vi "Value Change_Tools.vi"(8 "error in":errorcluster, 10 "NewVal":T8=enum."Ellipse", 11 "Data in":T1={"Class"={"Ants"=refnum, "Layer"=refnum, "Templates"=refnum, "Icon"=refnum, "Glyph"=refnum, "Settings"=refnum, "Tools"=refnum}, "Ref"={"Add Layer"=refnum, "Remove Layer"=refnum, "Line Text"=[], "Body Text Spec"=refnum, "DNL_Font"=refnum, "glyph path str"=refnum, "templates path str"=refnum, "Arrow Up"=refnum, "Arrow Down"=refnum, "IE VI Ref"=refnum, "Glyphs tree"=refnum, "Templates tree"=refnum, "Layer Icon Text"=refnum, "Layer Template"=refnum, "Clipboard"=refnum, "BW icon in"=refnum, "Color icon in"=refnum, "Layer Clust"=refnum, "Body Text"=refnum, "DNL_Framework Templates"=refnum, "Search Templates"=refnum, "TextMarker"=refnum, "Tab Control"=refnum, "Search Glyphs"=refnum, "Line Color"=refnum, "DNL_Glyphs []"=refnum, "Fill Color"=refnum, "Tools"=refnum, "Glyphs tree"=refnum, "Icon"=refnum, "Preview"=refnum, "Ants"=refnum, "Terminals"=refnum, "menu reference"=refnum, "LayerNames"=[], "GlyphLoadAnimation"=refnum, "TemplateLoadAnimation"=refnum, "refreshGlyphs"=refnum, "refreshTemplates"=refnum}, "Support"={"AntsRect"={"left"=0, "top"=0, "right"=0, "bottom"=0}, "Mouse Move Coords"={"Horizontal"=0, "Vertical"=0}, "Mouse Down Coords"={"Horizontal"=0, "Vertical"=0}, "Temp Coord"={"Horizontal"=0, "Vertical"=0}, "Action"=enum."Default", "Edge Color"=4914962, "Fill Color"=16860, "Mouse Down?"=FALSE, "Draft Mode?"=FALSE, "Temp Icon"=bytes[3102], "CTRL Pressed"=FALSE, "Move Selection?"=FALSE, "AntsRect Orig"={"left"=0, "top"=0, "right"=0, "bottom"=0}, "Text"="", "TM Set?"=FALSE, "Mouse inside icon?"=FALSE, "Tool (old value)"=0, "Pencil Move Color"=0, "Swap Colors?"=FALSE, "Shift pressed?"=FALSE}}) -> (0 "error out":errorcluster, 3 "Data out":T1={"Class"={"Ants"=refnum, "Layer"=refnum, "Templates"=refnum, "Icon"=refnum, "Glyph"=refnum, "Settings"=refnum, "Tools"=refnum}, "Ref"={"Add Layer"=refnum, "Remove Layer"=refnum, "Line Text"=[], "Body Text Spec"=refnum, "DNL_Font"=refnum, "glyph path str"=refnum, "templates path str"=refnum, "Arrow Up"=refnum, "Arrow Down"=refnum, "IE VI Ref"=refnum, "Glyphs tree"=refnum, "Templates tree"=refnum, "Layer Icon Text"=refnum, "Layer Template"=refnum, "Clipboard"=refnum, "BW icon in"=refnum, "Color icon in"=refnum, "Layer Clust"=refnum, "Body Text"=refnum, "DNL_Framework Templates"=refnum, "Search Templates"=refnum, "TextMarker"=refnum, "Tab Control"=refnum, "Search Glyphs"=refnum, "Line Color"=refnum, "DNL_Glyphs []"=refnum, "Fill Color"=refnum, "Tools"=refnum, "Glyphs tree"=refnum, "Icon"=refnum, "Preview"=refnum, "Ants"=refnum, "Terminals"=refnum, "menu reference"=refnum, "LayerNames"=[], "GlyphLoadAnimation"=refnum, "TemplateLoadAnimation"=refnum, "refreshGlyphs"=refnum, "refreshTemplates"=refnum}, "Support"={"AntsRect"={"left"=0, "top"=0, "right"=0, "bottom"=0}, "Mouse Move Coords"={"Horizontal"=0, "Vertical"=0}, "Mouse Down Coords"={"Horizontal"=0, "Vertical"=0}, "Temp Coord"={"Horizontal"=0, "Vertical"=0}, "Action"=enum."Default", "Edge Color"=4914962, "Fill Color"=16860, "Mouse Down?"=FALSE, "Draft Mode?"=FALSE, "Temp Icon"=bytes[3102], "CTRL Pressed"=FALSE, "Move Selection?"=FALSE, "AntsRect Orig"={"left"=0, "top"=0, "right"=0, "bottom"=0}, "Text"="", "TM Set?"=FALSE, "Mouse inside icon?"=FALSE, "Tool (old value)"=0, "Pencil Move Color"=0, "Swap Colors?"=FALSE, "Shift pressed?"=FALSE}})   [LabVIEW 2021]
uses:
  <resource>/plugins/NIIconEditor/Controls/Tools.ctl
  <resource>/plugins/NIIconEditor/Controls/Pen.ctl
  <resource>/plugins/NIIconEditor/Controls/Line.ctl
  <resource>/plugins/NIIconEditor/Controls/Dropper.ctl
  <resource>/plugins/NIIconEditor/Controls/Fill.ctl
  <resource>/plugins/NIIconEditor/Controls/IERect.ctl
  <resource>/plugins/NIIconEditor/Controls/FRect.ctl
  <resource>/plugins/NIIconEditor/Controls/Circle.ctl
  <resource>/plugins/NIIconEditor/Controls/FCircle.ctl
  <resource>/plugins/NIIconEditor/Controls/Rubber.ctl
  <resource>/plugins/NIIconEditor/Controls/Text.ctl
  <resource>/plugins/NIIconEditor/Controls/Selection.ctl
  <resource>/plugins/NIIconEditor/Controls/Move.ctl
  <resource>/plugins/NIIconEditor/Controls/IE Data.ctl
  <resource>/plugins/NIIconEditor/Class/Ants/Ants.lvclass
  <resource>/plugins/NIIconEditor/Class/FakedArray/FakedArray.lvclass
  <resource>/plugins/NIIconEditor/Class/Icon Library/Glyph.lvclass
  <resource>/plugins/NIIconEditor/Class/Settings/Settings.lvclass
  <resource>/plugins/NIIconEditor/Class/Tools/Tools Paint.lvclass
  <vilib>/LabVIEW Icon API/lv_icon/Classes/Icon/Icon.lvclass
  <resource>/plugins/NIIconEditor/Controls/IE Classes.ctl
  <resource>/plugins/NIIconEditor/Controls/References Cluster.ctl
  <resource>/plugins/NIIconEditor/Controls/SupportClass.ctl
  <vilib>/Utility/miscctls.llb/LVPoint32TypeDef.ctl
  <resource>/plugins/NIIconEditor/Controls/SupportClass_Action.ctl
  <vilib>/LabVIEW Icon API/lv_icon/Controls/IEColor.ctl
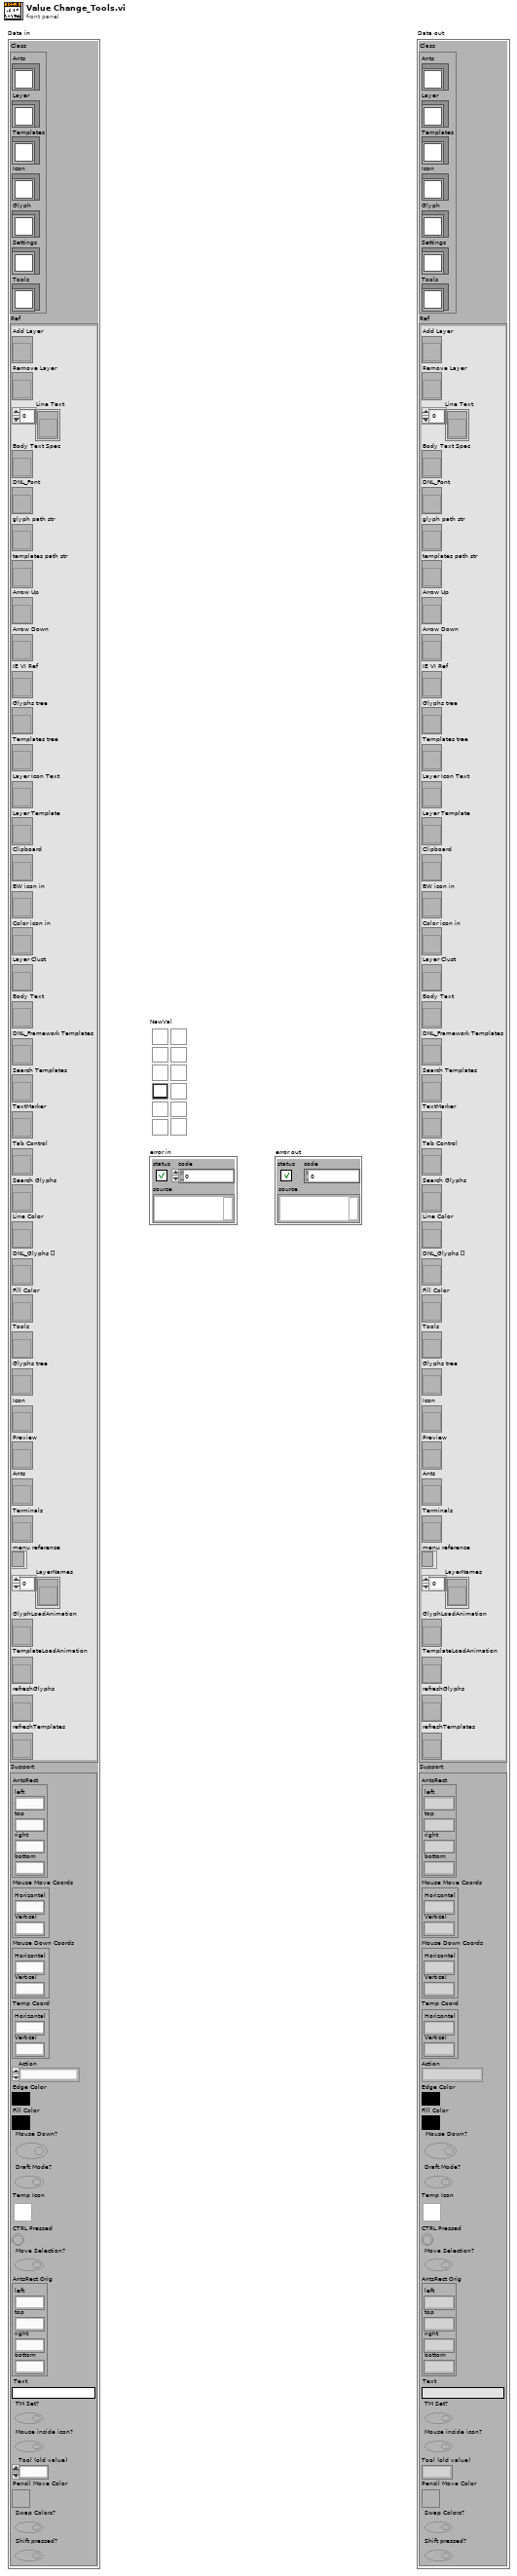
[diagram p1: front panel]
types:
  T1 = typedef "IE Data.ctl" = cluster{"Class":T2, "Ref":T3, "Support":T4}
  T2 = typedef "IE Classes.ctl" = cluster{"Ants":refnum<class "Ants.lvclass">, "Layer":refnum<class "FakedArray.lvclass">, "Templates":refnum<class "FakedArray.lvclass">, "Icon":refnum<class "Icon.lvclass">, "Glyph":refnum<class "Glyph.lvclass">, "Settings":refnum<class "Settings.lvclass">, "Tools":refnum<class "Tools Paint.lvclass">}
  T3 = typedef "References Cluster.ctl" = cluster{"Add Layer":refnum<vi>, "Remove Layer":refnum<vi>, "Line Text":refnum<vi>[], "Body Text Spec":refnum<vi>, "DNL_Font":refnum<vi>, "glyph path str":refnum<vi>, "templates path str":refnum<vi>, "Arrow Up":refnum<vi>, "Arrow Down":refnum<vi>, "IE VI Ref":refnum<vi>, "Glyphs tree":refnum<vi>, "Templates tree":refnum<vi>, "Layer Icon Text":refnum<vi>, "Layer Template":refnum<vi>, "Clipboard":refnum<vi>, "BW icon in":refnum<vi>, "Color icon in":refnum<vi>, "Layer Clust":refnum<vi>, "Body Text":refnum<vi>, "DNL_Framework Templates":refnum<vi>, "Search Templates":refnum<vi>, "TextMarker":refnum<vi>, "Tab Control":refnum<vi>, "Search Glyphs":refnum<vi>, "Line Color":refnum<vi>, "DNL_Glyphs []":refnum<vi>, "Fill Color":refnum<vi>, "Tools":refnum<vi>, "Glyphs tree":refnum<vi>, "Icon":refnum<vi>, "Preview":refnum<vi>, "Ants":refnum<vi>, "Terminals":refnum<vi>, "menu reference":refnum<k9>, "LayerNames":refnum<vi>[], "GlyphLoadAnimation":refnum<vi>, "TemplateLoadAnimation":refnum<vi>, "refreshGlyphs":refnum<vi>, "refreshTemplates":refnum<vi>}
  T4 = typedef "SupportClass.ctl" = cluster{"AntsRect":cluster{"left":i16, "top":i16, "right":i16, "bottom":i16}, "Mouse Move Coords":T5, "Mouse Down Coords":T5, "Temp Coord":T5, "Action":T6, "Edge Color":T7, "Fill Color":T7, "Mouse Down?":bool, "Draft Mode?":bool, "Temp Icon":picture, "CTRL Pressed":bool, "Move Selection?":bool, "AntsRect Orig":cluster{"left":i16, "top":i16, "right":i16, "bottom":i16}, "Text":string, "TM Set?":bool, "Mouse inside icon?":bool, "Tool (old value)":u32, "Pencil Move Color":u32, "Swap Colors?":bool, "Shift pressed?":bool}
  T5 = typedef "LVPoint32TypeDef.ctl" = cluster{"Horizontal":i32, "Vertical":i32}
  T6 = typedef "SupportClass_Action.ctl" = enum16{"Default", "Move Selection", "Glyph Library", "Tool"}
  T7 = typedef "IEColor.ctl" = u32
  T8 = typedef "Tools.ctl" = enum32{"Pencil", "Line", "Dropper", "Fill", "Rectangle", "Filled Rectangle", "Ellipse", "Filled Ellipse", "Eraser", "Text", "Select", "Move"}
  T9 = cluster{"Horizontal":i32, "Vertical":i32, "Vertical 2":i32, "Vertical 3":i32}
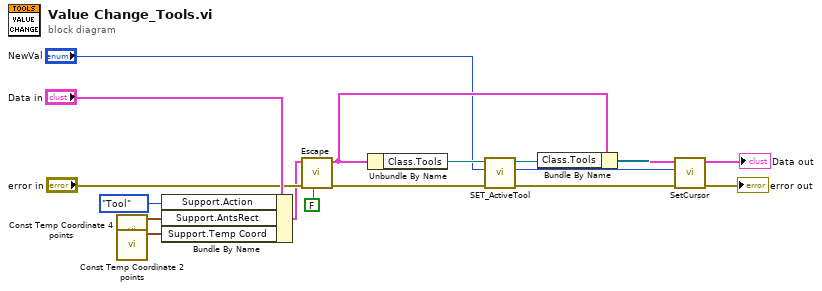
[diagram p0: block diagram]
diagram:
  n1 = call <resource>:"Const Temp Coordinate 4 points.vi"() -> ("Const Temp Coordinate"=w14:T9)  [unwired: 11 out]
  n2 = call <resource>:"Const Temp Coordinate 2 points.vi"() -> ("Const Temp Coordinate"=w16:T5)  [unwired: 11 out]
  n3 = Bundle By Name(cluster="Data in", "Support.Action"=SupportClass_Action."Tool" ("Action"), "Support.AntsRect"=w14, "Support.Temp Coord"=w16) -> (w11:T1)
  n4 = call <resource>:"Escape.vi"("Reset cursor (T)"=FALSE ("Reset cursor? (T)"), "error in"="error in", "Data in"=w11) -> ("error out"=w1:errorcluster, "Data out"=w9:T1)  [unwired: 1 in, 6 out]
  n5 = Unbundle By Name(w9) -> ("Class.Tools"=w10:refnum<class "Tools Paint.lvclass">)
  n6 = call-dynamic "SET_ActiveTool.vi"("error in (no error)"=w1, "Radio Buttons"="NewVal", "Tools Paint.lvclass in"=w10) -> ("error out"=w4:errorcluster, "Tools Paint.lvclass out"=w8:refnum<class "Tools Paint.lvclass">)  [unwired: 7 out]
  n7 = Bundle By Name(cluster=w9, "Class.Tools"=w8) -> (w7:T1)
  n8 = call <resource>:"SetCursor.vi"("error in (no error)"=w4, "Radio Buttons"="NewVal", "Data in"=w7) -> ("error out"=→"error out":errorcluster, "Data out"=→"Data out":T1)  [unwired: 7 out]
